vi "IVA Match Geometric Pattern Algorithm No advanced options.vi"(7 "Template":T1, 8 "error in (no error)":errorcluster, 9 "Settings":T5={"Curve Parameters"={"Extraction Mode"=0, "Edge Threshold"=30, "Edge Filter Size"=1, "Min Length"=25, "Row Search Step Size"=5, "Col Search Step Size"=2, "Max Endpoint Gap"=10, "Closed"=FALSE, "Subpixel"=FALSE}, "Match Mode"={"Rotation"=TRUE, "Scale"=FALSE, "Occlusion"=FALSE, "Reserved"=FALSE, "Reserved"=FALSE, "Reserved"=FALSE}, "Range Settings"=[], "Number of Matches Requested"=1, "Minimum Match Score"=800.0, "Subpixel Accuracy"=FALSE} {"Minimum Match Score" min=0 max=1000 format="%.2f"; "Number of Matches Requested" min=1; "Range Settings"."Max" format="%.2f"; "Range Settings"."Min" format="%.2f"; "Range Settings"."Match Constraints" items=["Rotation Angle (degrees)", "Scale Factor (%)", "Occlusion (%)"]; "Curve Parameters"."Extraction Mode" items=["Normal", "Uniform Regions"]; "Curve Parameters"."Edge Filter Size" items=["Fine", "Normal", "Contour Tracing"]; "Curve Parameters"."Max Endpoint Gap" min=0; "Curve Parameters"."Col Search Step Size" min=1 max=255 step=1; "Curve Parameters"."Row Search Step Size" min=1 max=255 step=1; "Curve Parameters"."Min Length" min=0; "Curve Parameters"."Edge Threshold" min=1 max=350 step=1}, 10 "ROI Descriptor":T6 {"Contours"."Type" items=["No Selection", "Point", "Line", "Rectangle", "Oval", "Polygon", "Freehand Region", "Annulus", "Unused2", "Unused3", "Broken Line", "Freehand Line", "Rotated Rectangle"]}, 11 "Image":T1) -> (0 "error out":errorcluster, 1 "Calibrated Matches":T2[](array[typedef]) {"Correlation Score" format="%.2f"; "Target Template Curve Score" format="%.2f"; "Template Target Curve Score" format="%.2f"; "Bounding Box"."y" format="%.2f"; "Bounding Box"."x" format="%.2f"; "Position"."y" format="%.2f"; "Position"."x" format="%.2f"; "Score" format="%.2f"; "Scale" format="%.2f"; "Angle" format="%.2f"; "Occlusion %" format="%.2f"}, 2 "Matches":T2[](array[typedef]) {"Correlation Score" format="%.2f"; "Target Template Curve Score" format="%.2f"; "Template Target Curve Score" format="%.2f"; "Bounding Box"."y" format="%.2f"; "Bounding Box"."x" format="%.2f"; "Position"."y" format="%.2f"; "Position"."x" format="%.2f"; "Score" format="%.2f"; "Scale" format="%.2f"; "Angle" format="%.2f"; "Occlusion %" format="%.2f"}, 5 "Number of Matches":i32)   [LabVIEW 2011]
uses:
  <vilib>/vision/Pattern Matching.llb/IMAQ GM Match Report.ctl
  <vilib>/vision/Image Controls.llb/IMAQ Image.ctl
  <vilib>/vision/Pattern Matching.llb/IMAQ Curve Parameters.ctl
  <vilib>/vision/Pattern Matching.llb/IMAQ Match Range Setting.ctl
  <vilib>/vision/NI_Vision_Development_Module.lvlib
panel:
  # "Range"
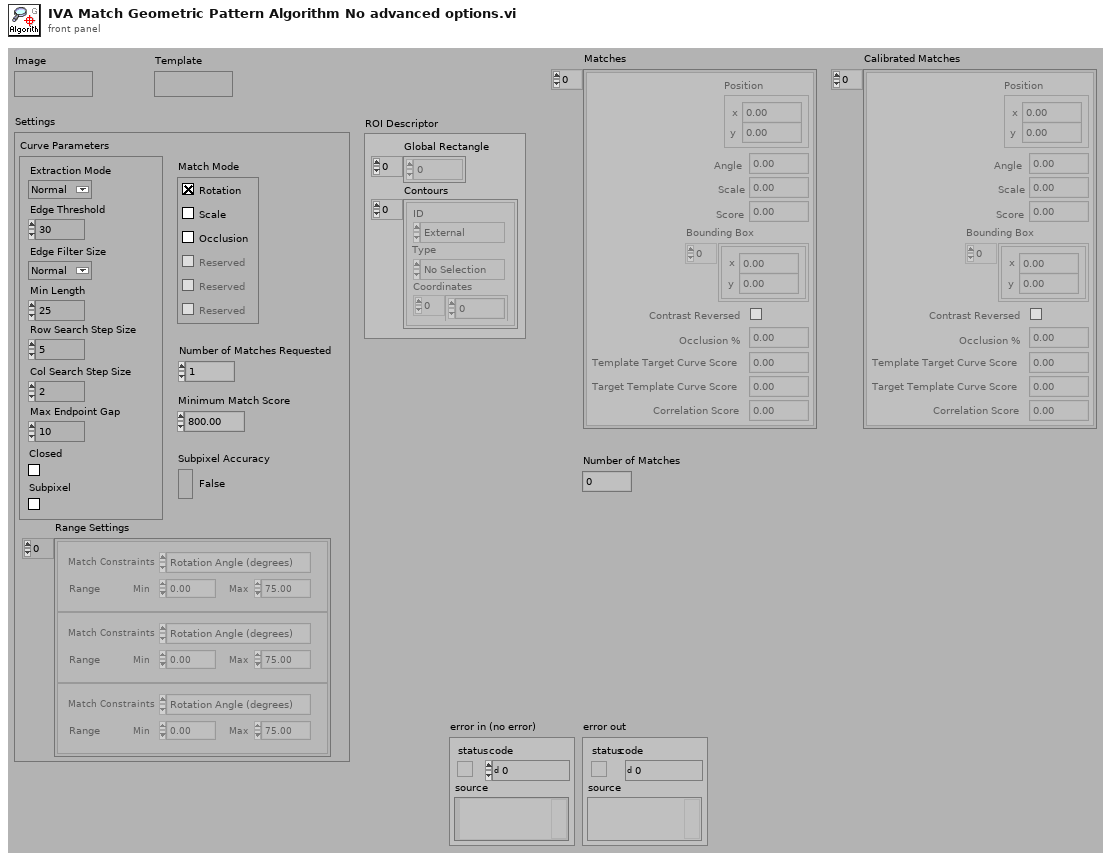
[diagram p1: front panel]
types:
  T1 = typedef "IMAQ Image.ctl" = refnum<image>
  T2 = typedef "IMAQ GM Match Report.ctl" = cluster{"Position":cluster{"x":sgl, "y":sgl}, "Angle":sgl, "Scale":sgl, "Score":sgl, "Bounding Box":cluster{"x":sgl, "y":sgl}[], "Contrast Reversed":bool, "Occlusion %":sgl, "Template Target Curve Score":sgl, "Target Template Curve Score":sgl, "Correlation Score":sgl}
  T3 = typedef "IMAQ Curve Parameters.ctl" = cluster{"Extraction Mode":u32, "Edge Threshold":i32, "Edge Filter Size":u32, "Min Length":i32, "Row Search Step Size":i32, "Col Search Step Size":i32, "Max Endpoint Gap":i32, "Closed":bool, "Subpixel":bool}
  T4 = typedef "IMAQ Match Range Setting.ctl" = cluster{"Match Constraints":u32, "Min":dbl, "Max":dbl}
  T5 = cluster{"Curve Parameters":T3, "Match Mode":cluster{"Rotation":bool, "Scale":bool, "Occlusion":bool, "Reserved":bool, "Reserved":bool, "Reserved":bool}, "Range Settings":T4[], "Number of Matches Requested":i32, "Minimum Match Score":sgl, "Subpixel Accuracy":bool}
  T6 = cluster{"Global Rectangle":i32[], "Contours":cluster{"ID":enum32{"External", "Internal"}, "Type":u32, "Coordinates":i32[]}[]}
  T7 = cluster{"Rotation":bool, "Scale":bool, "Occlusion":bool, "Reserved":bool, "Reserved":bool, "Reserved":bool}
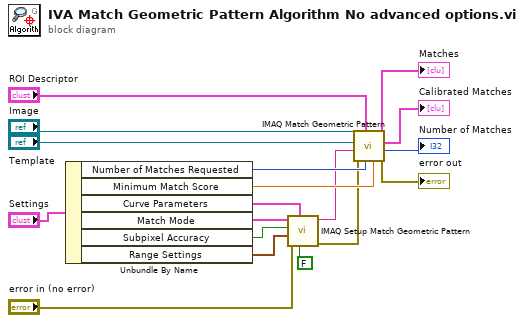
[diagram p0: block diagram]
diagram:
  n1 = Unbundle By Name("Settings") -> ("Number of Matches Requested"=w3:i32, "Minimum Match Score"=w4:sgl, "Curve Parameters"=w14:T3, "Match Mode"=w18:T7, "Subpixel Accuracy"=w15:bool, "Range Settings"=w16:T4[])
  n2 = call "IMAQ Setup Match Geometric Pattern"("Use Learn Curve Parameters"=FALSE, "Curve Parameters"=w14, "error in (no error)"="error in (no error)", "Range Settings"=w16, "Subpixel Accuracy"=w15, "Match Mode"=w18) -> ("error out"=w2:errorcluster, "Match Geometric Pattern Setup Data"=w1:string)  [unwired: 4 out]
  n3 = call "IMAQ Match Geometric Pattern"("Minimum Match Score"=w4, "Number of Matches Requested"=w3, "ROI Descriptor"="ROI Descriptor", "error in (no error)"=w2, "Match Geometric Pattern Setup Data"=w1, "Template Image"="Template", "Image"="Image") -> ("error out"=→"error out":errorcluster, "Number of Matches"=→"Number of Matches":i32, "Matches (real-world)"=→"Calibrated Matches":T2[], "Matches (pixel)"=→"Matches":T2[])  [unwired: 1 out]
